vi "CSM Check - StateType.vi"(8 "Matched Previous?":bool, 10 "Cross CSM Data (in)":T1={"Name(\"\" to use uuid)"="", "Current State"="", "Arguments"="", "Source Message"={"‘State"="", "’Arguments"="", "’Error"={"status"=FALSE, "code"=0, "source"=""}}, "Source Module"="", "Complete(T)/Start(F)"=FALSE, "LogType"=enum."State Change"}, 11 "GlobalLogFilter.lvclass":refnum<class "LogFilter.lvclass">) -> (0 "Matched? (dup)":bool, 2 "Cross CSM Data":T1={"Name(\"\" to use uuid)"="", "Current State"="", "Arguments"="", "Source Message"={"‘State"="", "’Arguments"="", "’Error"={"status"=FALSE, "code"=0, "source"=""}}, "Source Module"="", "Complete(T)/Start(F)"=FALSE, "LogType"=enum."State Change"}, 3 "GlobalLogFilter.lvclass (dup)":refnum<class "LogFilter.lvclass">)   [LabVIEW 2020, in "Communicable State Machine.lvlib" / "LogFilter.lvclass"]
uses:
  LogFilter.lvclass
  _CSM_GlobalLog_MSG.ctl
  _CSM_Response Source Message.ctl
  _CSM_GlobalLog_MSG_TYPE.ctl
  LogFilter.lvclass/LogFilter.ctl
  _CSM_GlobalLog_STATE_TYPE.ctl
  Communicable State Machine.lvlib
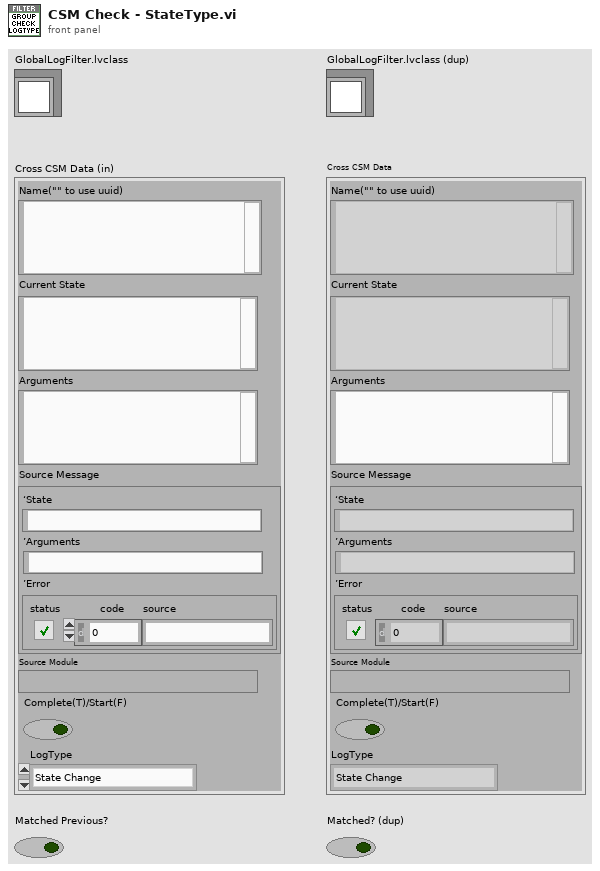
[diagram p1: front panel]
types:
  T1 = typedef "Communicable State Machine.lvlib/_CSM_GlobalLog_MSG.ctl" = cluster{"Name(\"\" to use uuid)":string, "Current State":string, "Arguments":string, "Source Message":T2, "Source Module":string, "Complete(T)/Start(F)":bool, "LogType":T3}
  T2 = typedef "Communicable State Machine.lvlib/_CSM_Response Source Message.ctl" = cluster{"‘State":string, "’Arguments":string, "’Error":errorcluster}
  T3 = typedef "Communicable State Machine.lvlib/_CSM_GlobalLog_MSG_TYPE.ctl" = enum16{"User Log", "State Change", "Status", "Interrupt", "Register", "Unregister", "Error Log", "Module Created", "Module Destroyed"}
  T4 = typedef "Communicable State Machine.lvlib/_CSM_GlobalLog_STATE_TYPE.ctl" = enum16{"State - Internal State", "State - External Message", "State - Response", "State - Complete"}
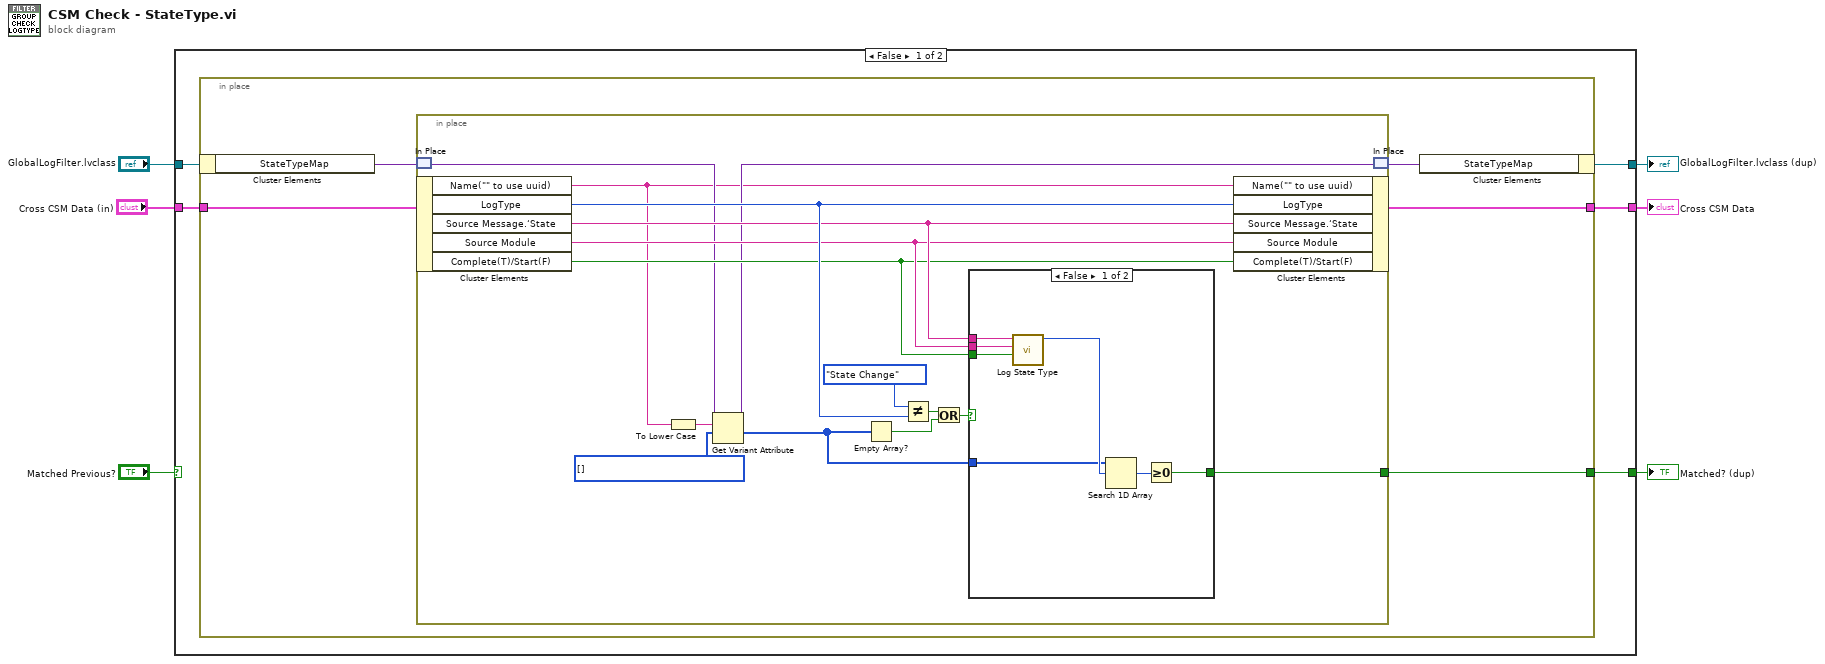
[diagram p0: block diagram]
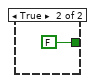
[diagram p2: hidden frame]
diagram:
  n1 = case shown="False" "Matched Previous?" {
    selector: "Matched Previous?" -> [_ w41]
    tunnel: [w10 w42] -> w5
    tunnel: "Cross CSM Data (in)" -> [w11 w42]
    tunnel: [w9 w41] -> w3
    tunnel: [w7 w40] -> w2
    tunnel: "GlobalLogFilter.lvclass" -> [w8 w40]
    frame False {
      n2 = in-place {
        in-place-border: w11 -> [w16]
        in-place-border: [w15] -> w10
        in-place-border: [w14] -> w9
        n3 = in-place-cluster #1(w8) -> ("StateTypeMap"=w13:variant)
        n4 = in-place {
          in-place-border: [w31] -> w14
          w18 = T4[] [] items=["State - Internal State", "State - External Message", "State - Response", "State - Complete"] ("Array")
          n5 = in-place-match #2(w13) -> (w22:variant)
          n6 = in-place-cluster #3(w16) -> ("Name(\"\" to use uuid)"=w20:string, "LogType"=w30:T3, "Source Message.‘State"=w25:string, "Source Module"=w24:string, "Complete(T)/Start(F)"=w23:bool)
          n7 = To Lower Case(string=w20) -> (all lower case string=w19:string)
          n8 = Get Variant Attribute(Variant=w22, name=w19, default value (empty Variant)=w18) -> (duplicate Variant=w21:variant, value=w17:T4[])  [unwired: 1 in, 2 out]
          n9 = Empty Array?(array=w17) -> (empty?=w26:bool)
          n10 = Not Equal?(x=_CSM_GlobalLog_MSG_TYPE."State Change", y=w30) -> (x != y?=w27:bool)
          n11 = Or(x=w27, y=w26) -> (x .or. y?=w28:bool)
          n12 = case shown="False" w28 {
            tunnel: [w34 FALSE] -> w31
            tunnel: w25 -> [w36 _]
            tunnel: w24 -> [w37 _]
            tunnel: w23 -> [w38 _]
            tunnel: w17 -> [w32 _]
            frame False {
              n13 = call "Log State Type.vi"("Complete(T)/Start(F)"=w38, "Source Module"=w37, "‘State"=w36) -> ("CSM_GlobalLog_STATE_TYPE"=w33:T4)  [unwired: 8 in]
              n14 = Search 1D Array(1D array=w32, element=w33) -> (index of element=w35:i32)  [unwired: 1 in]
              n15 = Greater Or Equal To 0?(x=w35) -> (x >= 0?=w34:bool)
            }
            frame True {
            }
          }
          n16 = in-place-cluster #3("Name(\"\" to use uuid)"=w20, "LogType"=w30, "Source Message.‘State"=w25, "Source Module"=w24, "Complete(T)/Start(F)"=w23) -> (w15:T1)
          n17 = in-place-match #2(w21) -> (w12:variant)
        }
        n18 = in-place-cluster #1("StateTypeMap"=w12) -> (w7:refnum<class "LogFilter.lvclass">)
      }
    }
    frame True {
    }
  }
  "Cross CSM Data" <- w5
  "Matched? (dup)" <- w3
  "GlobalLogFilter.lvclass (dup)" <- w2
